vi "PXI-4132 Configure DCpwr (RT).vi"(8 "error in (no error)":errorcluster, 11 "Device Ref in":T1 format="%.0x") -> (0 "error out":errorcluster, 2 "Channel 0 Type":i32, 3 "Device Ref out":T1 format="%.0x", 4 "Defaults":dbl[](array[numeric]), 5 "instrument handle out":refnum<k15>, 6 "input FIFO Indexes":i32[](array[numeric]))   [LabVIEW 2013, in "PXI-4132 Custom Device.lvlib"]
uses:
  PXI-4132 Custom Device.lvlib
  <vilib>/NI Veristand/Custom Device API/Custom Device Item Ref.ctl
  <instrlib>/niDCPower/nidcpower.llb/niDCPower Source Mode.ctl
  PXI-4132 Global Variable.vi
  <vilib>/NI Veristand/Custom Device API/Get Item Property (String).vi
  <vilib>/NI Veristand/Custom Device API/Get Item Property (I32).vi
  <vilib>/NI VeriStand/Custom Device API/Custom Device API.lvlib
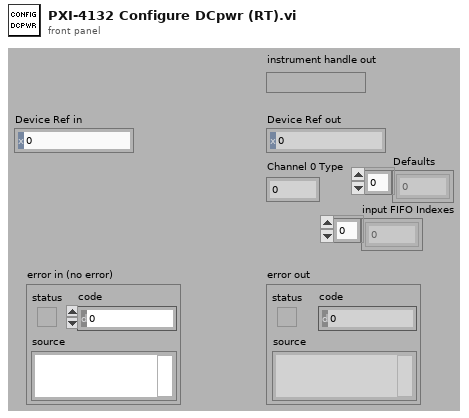
[diagram p1: front panel]
types:
  T1 = typedef "Custom Device API.lvlib/Custom Device Item Ref.ctl" = u64
  T2 = typedef "niDCPower Source Mode.ctl" = i32
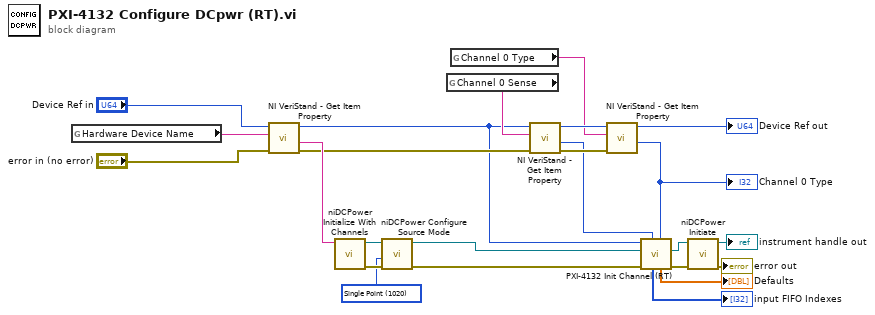
[diagram p0: block diagram]
diagram:
  w8 = T2 1020 items=["Single Point"=1020, "Sequence"=1021] ("source mode")
  n1 = global read "PXI-4132 Global Variable.vi" "Hardware Device Name"() -> (w24:string)
  n2 = call-poly <vilib>:"NI VeriStand - Get Item Property.vi"("error in (no error)"="error in (no error)", "Property Name"=w24, "Item Ref in"="Device Ref in") -> ("error out"=w21:errorcluster, "Value"=w23:string, "Item Ref out"=w14:T1)  [unwired: 5 in, 1 out]
  n3 = call <instrlib>:"niDCPower Initialize With Channels.vi"("resource name"=w23) -> ("error out"=w10:errorcluster, "instrument handle out"=w12:refnum<k15>)  [unwired: 9 in]
  n4 = call <instrlib>:"niDCPower Configure Source Mode.vi"("error in (no error)"=w10, "source mode"=w8, "instrument handle"=w12) -> ("error out"=w9:errorcluster, "instrument handle out"=w11:refnum<k15>)  [unwired: 7 in]
  n5 = global read "PXI-4132 Global Variable.vi" "Channel 0 Sense"() -> (w19:string)
  n6 = global read "PXI-4132 Global Variable.vi" "Channel 0 Type"() -> (w18:string)
  n7 = call-poly <vilib>:"NI VeriStand - Get Item Property.vi"("error in (no error)"=w21, "Property Name"=w19, "Item Ref in"=w14) -> ("error out"=w20:errorcluster, "Value"=w17:i32, "Item Ref out"=w22:T1)  [unwired: 5 in, 1 out]
  n8 = call-poly <vilib>:"NI VeriStand - Get Item Property.vi"("error in (no error)"=w20, "Property Name"=w18, "Item Ref in"=w22) -> ("Value"=w16:i32, "Item Ref out"=→"Device Ref out":T1)  [unwired: 5 in, 2 out]
  "Channel 0 Type" <- w16
  n9 = call "PXI-4132 Init Channel (RT).vi"("Channel Type"=w16, "Channel Sense"=w17, "error in (no error)"=w9, "resource name"=w11, "Device Reference In"=w14) -> ("error out"=w15:errorcluster, "resource name Out"=w13:refnum<k15>, "Defaults"=→"Defaults":dbl[], "FIFO Indexes"=→"input FIFO Indexes":i32[])  [unwired: 2 in, 1 out]
  n10 = call <instrlib>:"niDCPower Initiate.vi"("error in (no error)"=w15, "instrument handle"=w13) -> ("error out"=→"error out":errorcluster, "instrument handle out"=→"instrument handle out":refnum<k15>)  [unwired: 8 in]
